vi "E9_Local_Variable.vi"(10 "b":dbl, 11 "a":dbl) -> (9 "y":dbl)   [LabVIEW 2020]
panel:
  out "Ind Temp":dbl
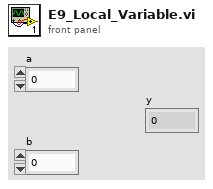
[diagram p1: front panel]
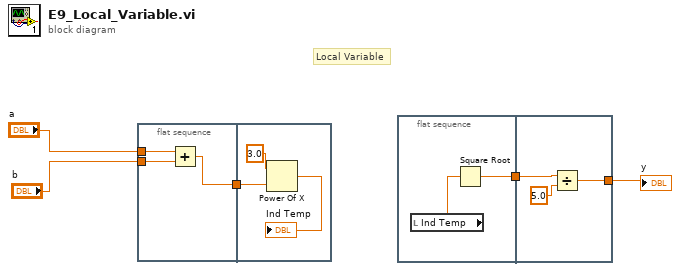
[diagram p0: block diagram]
diagram:
  # "Local Variable"
  n1 = flat-sequence {
    tunnel: "a" -> [w8]
    tunnel: "b" -> [w7]
    tunnel: [w6] -> w1
    tunnel: w1 -> [w9]
    frame #0 {
      n2 = Add(x=w8, y=w7) -> (x+y=w6:dbl)
    }
    frame #1 {
      n3 = Power Of X(1:w9, 2:3.0 ("y")) -> (0:→"Ind Temp":dbl)
    }
  }
  n4 = flat-sequence {
    tunnel: [w13] -> w3
    tunnel: w3 -> [w16]
    tunnel: [w14] -> w2
    frame #0 {
      n5 = local read "Ind Temp"() -> (w12:dbl)
      n6 = Square Root(x=w12) -> (sqrt(x)=w13:dbl)
    }
    frame #1 {
      n7 = Divide(x=w16, y=5.0) -> (x/y=w14:dbl)
    }
  }
  "y" <- w2
